vi "HealthAndStatusFIFOCopy.vi"(11 "HealthAndStatusSettingsFIFOCopySettings":T1={"InternalHealthAndStatusFIFO"="InternalHealthAndStatusFIFO", "SourceHealthAndStatusFIFO"="InternalHealthAndStatusFIFO"}) -> ()   [LabVIEW 2016, in "FPGAHealthAndStatus.lvlib"]
uses:
  FPGAHealthAndStatus.lvlib
  DataTypes/HealthAndStatusFIFOCopySettings.ctl
  <vilib>/rvi/Emulation/niFpgaGetClockAttributes.vi
  <vilib>/rvi/Emulation/niFpgaSctlEmulationGetInTimedLoop.vi
  <vilib>/rvi/Emulation/niFpgaEmulationReportErrorSimple.vi
  <vilib>/rvi/DataTransferAndStorage/Container/Common/niFpgaContainerExecOnDevCompGetState.vi
  <vilib>/rvi/Emulation/niFpgaEmulationIsFPGAContextNoSignature.vi
  <vilib>/rvi/errors/niFpgaSetErrorForExecOnDevCompSimple.vi
  <vilib>/rvi/eio/common/nirviEmuReportErrorAndStop.vi
  <vilib>/rvi/DataTransferAndStorage/Container/Common/niFpgaContainerGetUniqueNameForEmu.vi
  <vilib>/rvi/FIFO/Fifo_Resource/nirvififoEmulationSetSize.vi
  <vilib>/rvi/FIFO/Fifo_Resource/nirviFifoEmulationQueueMgr.vi
  <instcachedir>/0/nirviFifoEmulationQueueMgr_E5CAEC123FF24DC58D834DCA3CDAA9B5.lvgen/nirviFifoEmulationQueueMgr_E5CAEC123FF24DC58D834DCA3CDAA9B5_011.vi
  <vilib>/rvi/FIFO/Fifo_Resource/nirvififoEmulationDetermineInputValidOut.vi
  <vilib>/rvi/FIFO/Fifo_Resource/nirvififoEmulationCreateLock.vi
  <vilib>/rvi/Emulation/niFpgaProcessEmulError.vi
  <vilib>/rvi/FIFO/Fifo_Resource/nirvififoEmulationObtainLock.vi
  <vilib>/rvi/FIFO/Fifo_Resource/nirvififoEmulationReleaseLock.vi
  <vilib>/rvi/occurrence/nirviWaitOnOccurrenceBase.vi
  <vilib>/rvi/errors/nirviReportUnexpectedCaseInternalError.vi
  <vilib>/rvi/errors/nirviReportUnexpectedCaseInternalError (U32).vi
  <vilib>/Utility/error.llb/Clear Errors.vi
  <vilib>/rvi/interface/RandomDataEmulation/niFpgaRandomDataHandleErrors.vi
  <vilib>/rvi/Emulation/niFpgaCriticalErrorInLSC.vi
  <vilib>/rvi/DataTransferAndStorage/Container/XNode/niFpgaContainer.xnode
  <vilib>/rvi/FIFO/Fifo_Resource/niFpgaFifoEmulationRefIn.vi
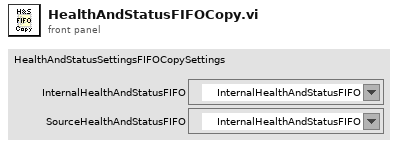
[diagram p1: front panel]
types:
  T1 = typedef "FPGAHealthAndStatus.lvlib/HealthAndStatusFIFOCopySettings.ctl" = cluster{"InternalHealthAndStatusFIFO":refnum<k21>, "SourceHealthAndStatusFIFO":refnum<k21>}
  T2 = cluster{"Address":u32, "UpdateMode":enum8{"NOP", "Set", "Add", "Subtract", "Or"}, "Data":u64}
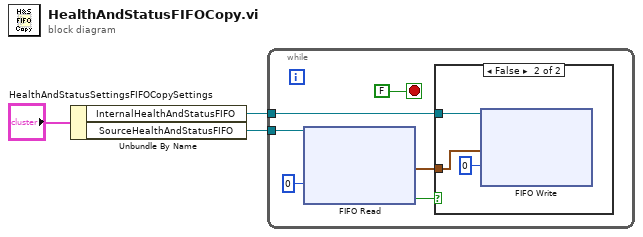
[diagram p0: block diagram]
diagram:
  n1 = Unbundle By Name("HealthAndStatusSettingsFIFOCopySettings") -> ("InternalHealthAndStatusFIFO"=w2:refnum<k21>, "SourceHealthAndStatusFIFO"=w1:refnum<k21>)
  n2 = while {
    tunnel: w2 -> [w5]
    tunnel: w1 -> [w8]
    stop <- FALSE stop-if-true
    n3 = xnode "FIFO Read"("Timeout"=0, "FIFO In"=w8) -> ("Element"=w4:T2, "Timed Out?"=w6:bool)  [unwired: 1 out]
    n4 = case shown="False" w6 {
      tunnel: w5 -> [_ w12]
      tunnel: w4 -> [_ w11]
      frame True {
      }
      frame False {
        n5 = xnode "FIFO Write"("Element"=w11, "Timeout"=0, "FIFO In"=w12) -> ()  [unwired: 2 out]
      }
    }
  }
